vi "SMU Measure.vi"(8 "error in (no error)":errorcluster, 10 "SMUSequenceNumberOfSteps":i32, 11 "IVI Refnum in":refnum<k15>) -> (0 "error out":errorcluster, 1 "Numeric":dbl, 2 "Numeric 2":dbl, 3 "IVI Refnum out":refnum<k15>, 4 "in compliance":bool[](array[boolean]))   [LabVIEW 2019, in "SupportVIs.lvlib"]
uses:
  SupportVIs.lvlib
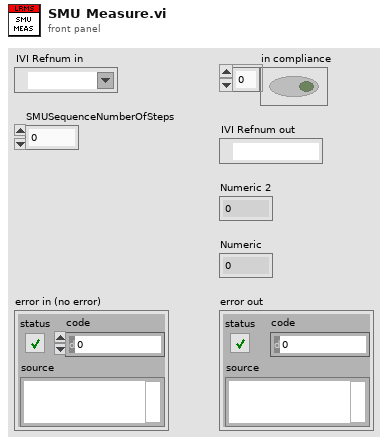
[diagram p1: front panel]
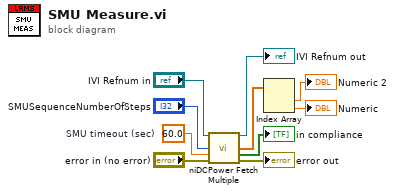
[diagram p0: block diagram]
diagram:
  w4 = 60.0  # SMU timeout (sec)
  n1 = call <instrlib>:"niDCPower Fetch Multiple.vi"("instrument handle"="IVI Refnum in", "count (1)"="SMUSequenceNumberOfSteps", "timeout (sec)"=w4, "error in (no error)"="error in (no error)") -> ("instrument handle out"=→"IVI Refnum out":refnum<k15>, "current measurements"=w8:dbl[], "in compliance"=→"in compliance":bool[], "error out"=→"error out":errorcluster)  [unwired: 6 in, 2 out]
  n2 = Index Array(array=w8) -> (element #1=→"Numeric 2":dbl, element #2=→"Numeric":dbl)  [unwired: 2 in]
